vi "SC2 RT.vi"() -> ()   [LabVIEW 2015]
uses:
  SC2 states.ctl
  <vilib>/Platform/TimedLoop/XDataNode/timing_clust.ctl
  <vilib>/Platform/TimedLoop/XDataNode/nitl_modes.ctl
  <vilib>/Platform/TimedLoop/XDataNode/wakeup.ctl
  Encoder bit cluster.ctl
  <vilib>/Platform/TimedLoop/XDataNode/loadnilvce.vi
  <vilib>/Motion/Express/_s/nimc.fb.straightLineMove.startStraightLineMove.axis.modeRelative.0.vi
  <vilib>/Platform/TimedLoop/XDataNode/XDataNode.xnode
  <vilib>/Motion/BlockNode/FB.NIMotion.xnode
  <vilib>/Platform/TimedLoop/XDataNode/XDNodeRunTimeDep.lvlib
  <vilib>/nisyscfg/nisyscfg.lvlib
  <vilib>/nisyscfg/Find Hardware.vi
panel:
  out "Encoder displacement":i32
  in  "Random Sample":bool
  out "Within window?":bool
  in  "Stop":bool
  out "Motor status":bool=TRUE
  in  "Encoder offset":i32=-1277
  in  "Start Sample Change":bool
  out "SC2 State Control":T1=enum."wait"
  out "Encoder readback":errorcluster
  in  "error in (no error)":errorcluster
  out "status":bool
  out "Encoder destination":i32
  in  "New Move (Motor steps)":dbl=10000.0 format="%#_13g"
  in  "New Sample":i16
  in  "Step Window radius":i32=2
  out "Converted Encoder":bool[](array[boolean])
  in  "Motion Resource":refnum<k21>="Axis 1"
  out "Straight Line Move":errorcluster
  out "Raw Encoder":bool[](array[boolean])
  out "Encoder rotation":u16(graph)
  out "Encoder Position":i32
  # "Encoder offset required to \n\"line up\" encoder with wheel.\nSample 64 is -1021 encoder steps\n (or +15362 steps) from the \nencoder's zero point.. Note: Sample \nand encoder numbering run in \nopposite directions"
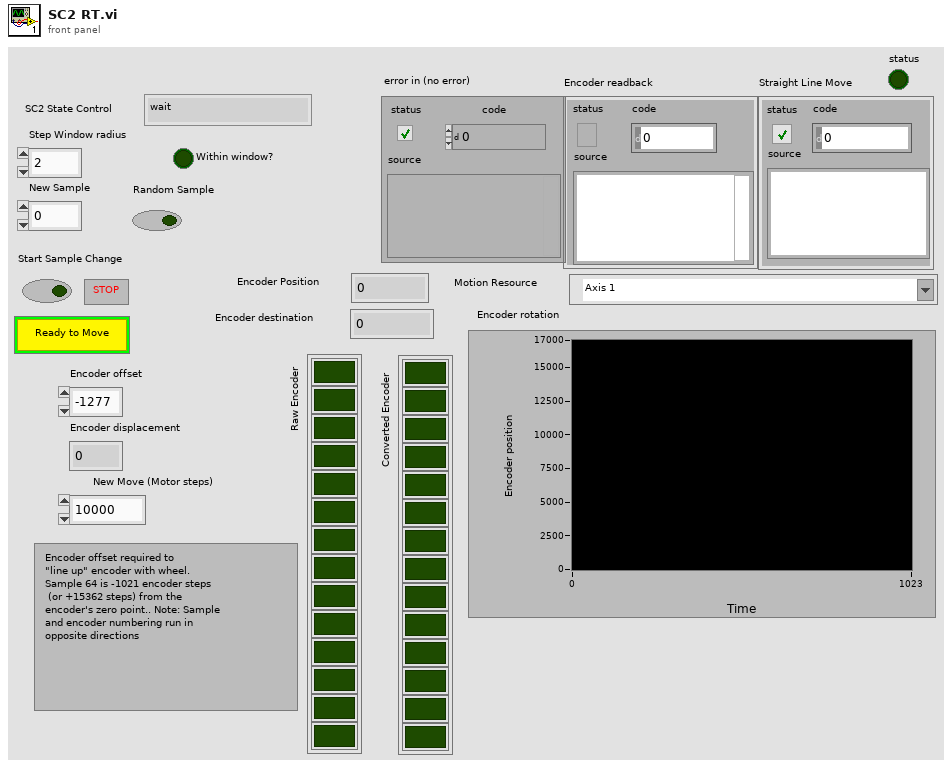
[diagram p1: front panel]
types:
  T1 = typedef "SC2 states.ctl" = enum16{"initialize", "wait", "check position", "rotate wheel", "rotate complete"}
  T2 = typedef "XDNodeRunTimeDep.lvlib/timing_clust.ctl" = cluster{"Expected End [f-1]":u64, "Actual End [f-1]":u64, "Finished Late? [f-1]":bool, "Expected End [i-1]":u64, "Actual End [i-1]":u64, "Finished Late? [i-1]":bool, "Expected Start [i]":u64, "Actual Start [i]":u64, "Expected Start [f]":u64, "Actual Start [f]":u64, "Source Name":string, "Structure Name":string, "Period":i64, "Deadline":i64, "Offset":i64, "Start":i64, "Priority":i32, "Timeout":i32, "Mode":T3, "Wakeup Reason":T4, "Error":errorcluster, "Source Type":string, "Secondary Source Type":string, "Global End Time":u64, "Global Start Time":u64, "Frame Duration":u64, "Iteration Duration":u64, "Assigned CPU":i32, "I/O Scan Engine Mode":u32}
  T3 = typedef "XDNodeRunTimeDep.lvlib/nitl_modes.ctl" = enum32{"No Change", "Process missed periods, maintain original phase", "Discard missed periods, maintain original phase", "Process missed periods, ignore original phase", "Discard missed periods, ignore original phase"}
  T4 = typedef "XDNodeRunTimeDep.lvlib/wakeup.ctl" = enum32{"Normal", "Aborted", "Asynchronous wakeup", "Timing source error", "Timed loop error", "Timeout"}
  T5 = typedef "Encoder bit cluster.ctl" = cluster{"MSB":bool, "13th bit":bool, "12th bit":bool, "11th bit":bool, "10th bit":bool, "9th bit":bool, "8th bit":bool, "7th bit":bool, "6th bit":bool, "5th bit":bool, "4th bit":bool, "3rd bit":bool, "2nd bit":bool, "LSB":bool}
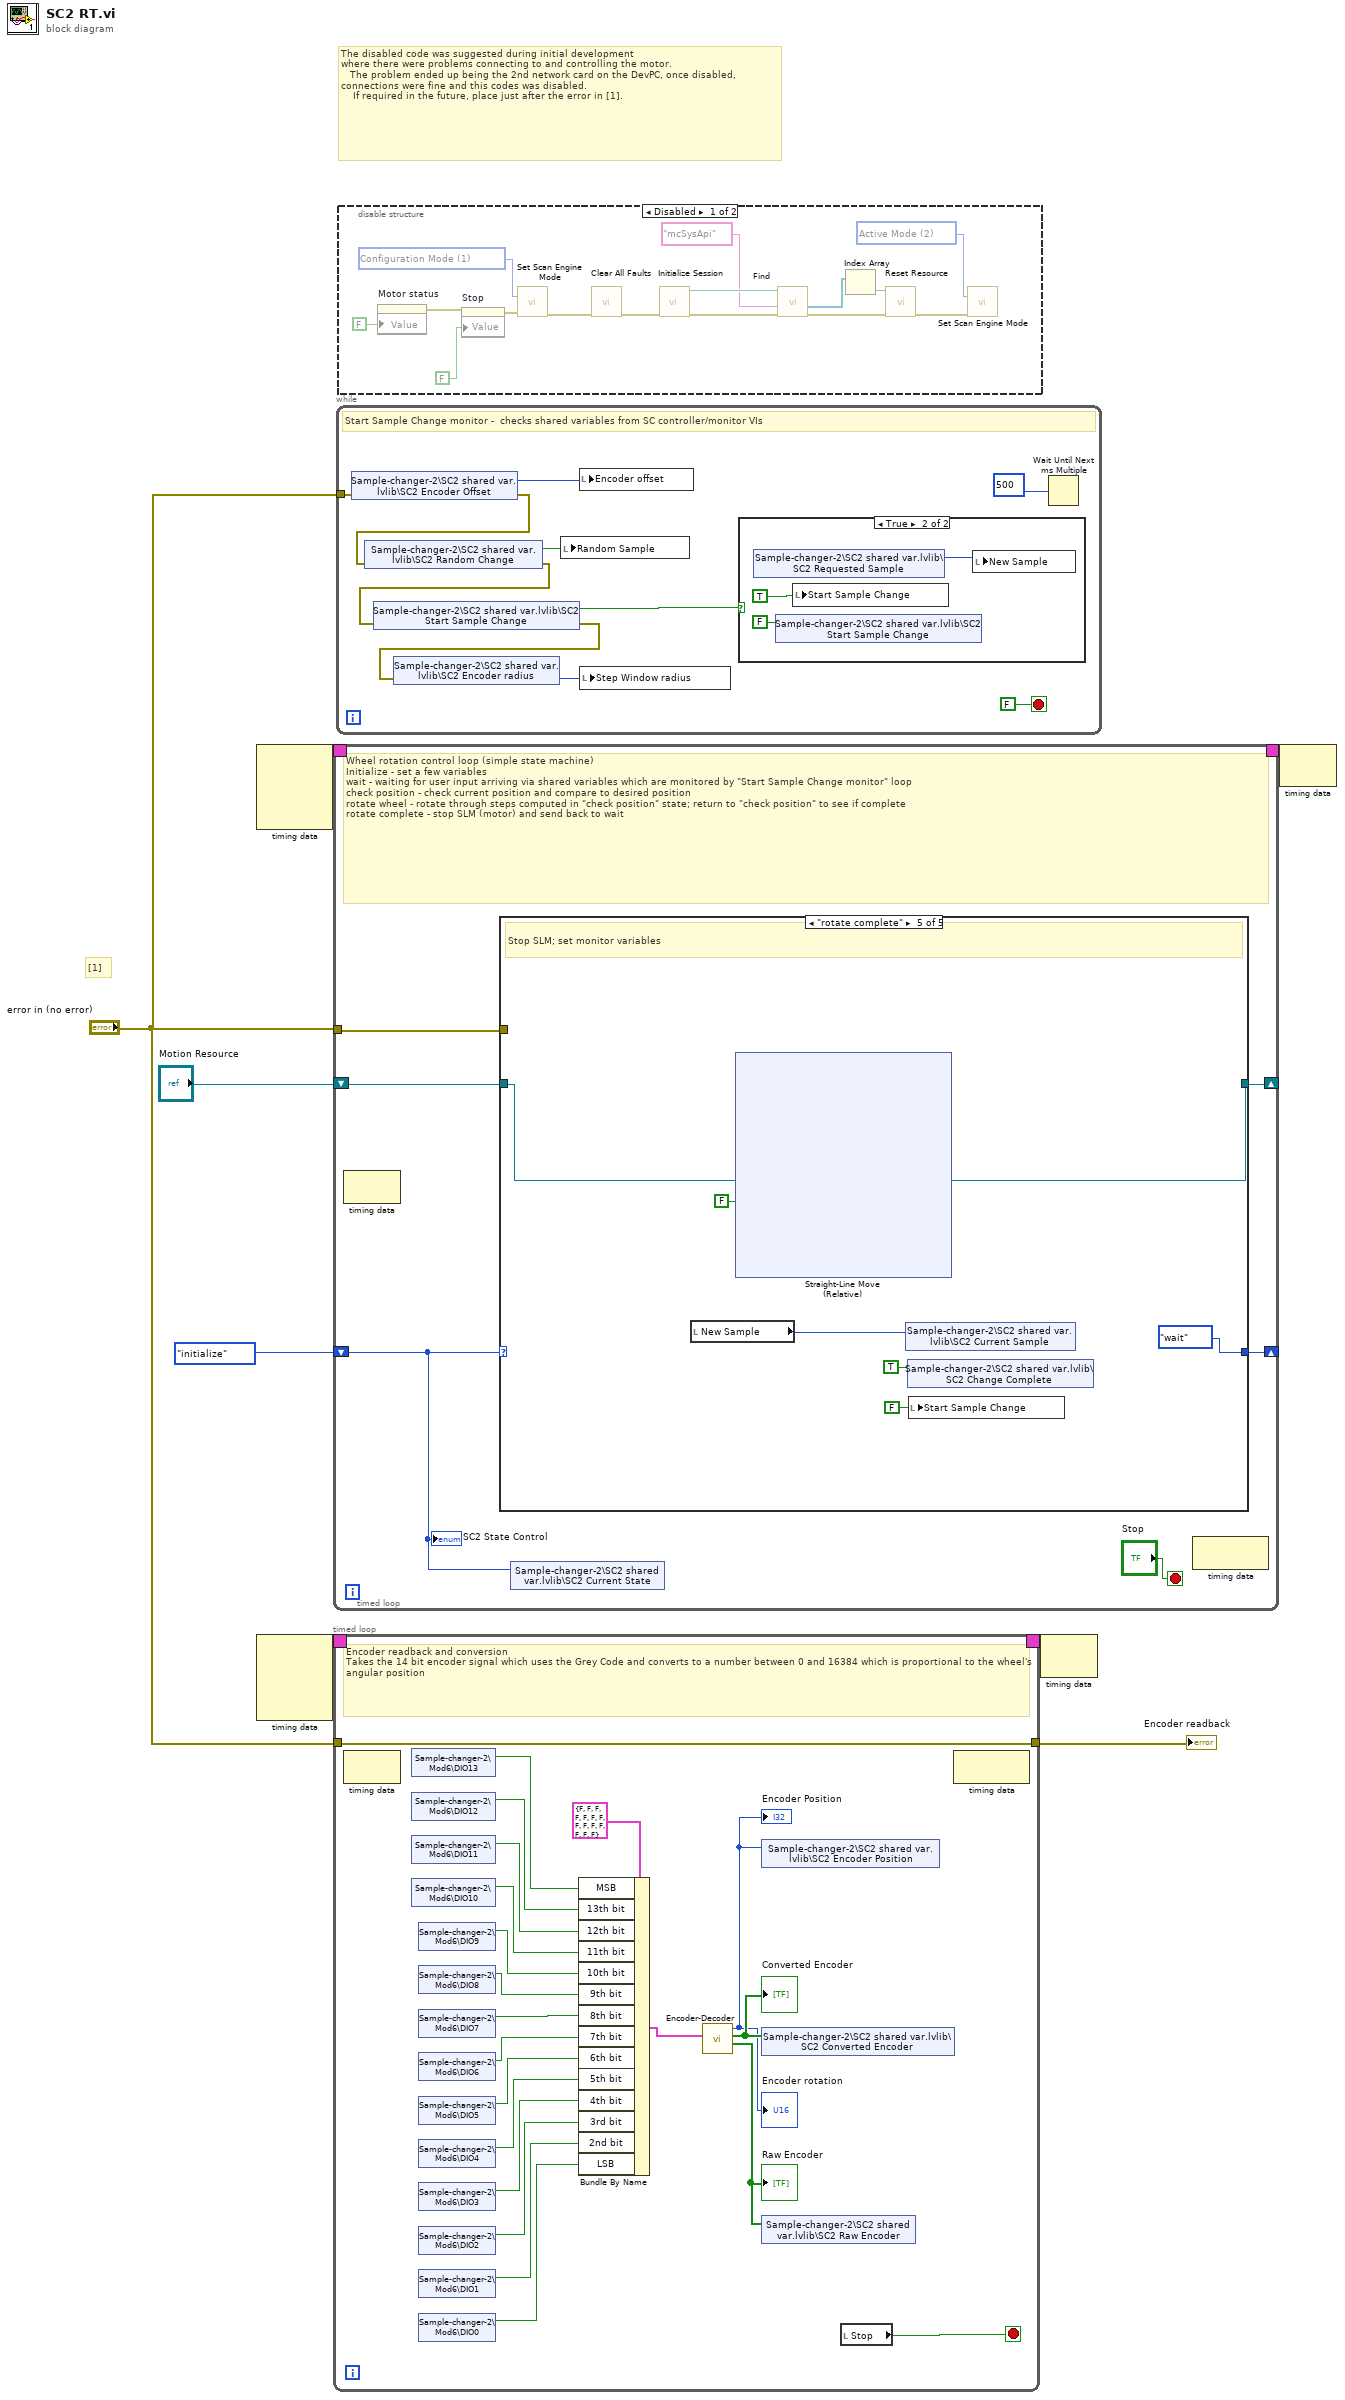
[diagram p0: block diagram]
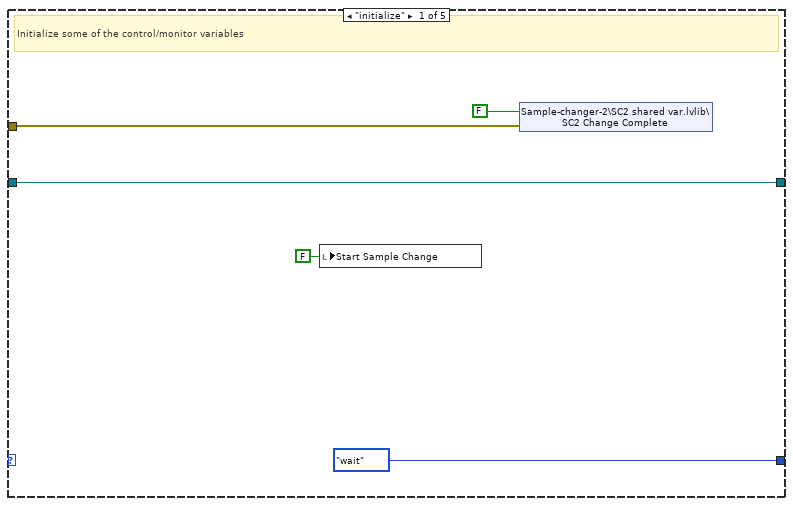
[diagram p4: hidden frame]
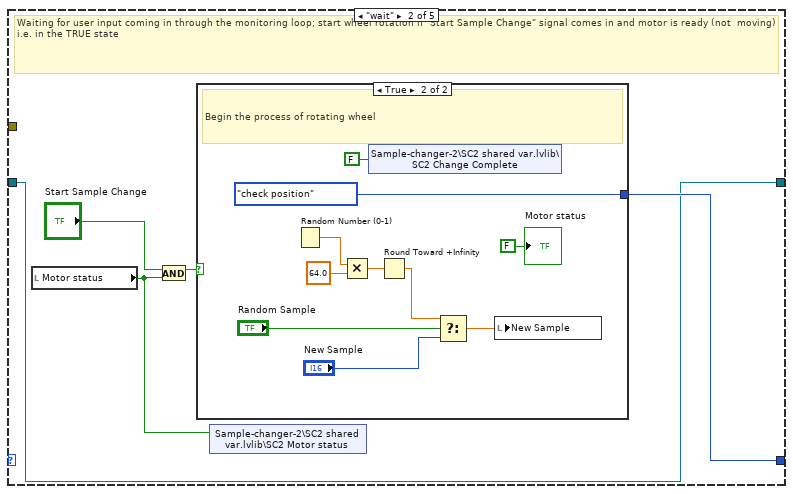
[diagram p5: hidden frame]
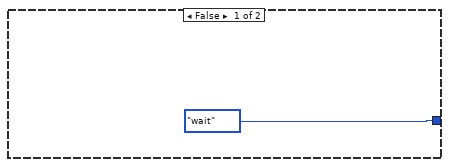
[diagram p6: hidden frame]
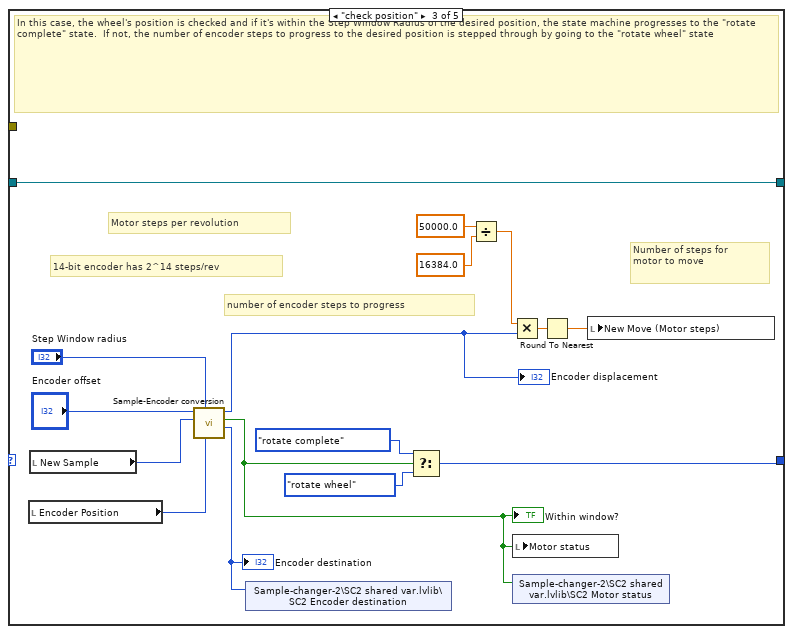
[diagram p7: hidden frame]
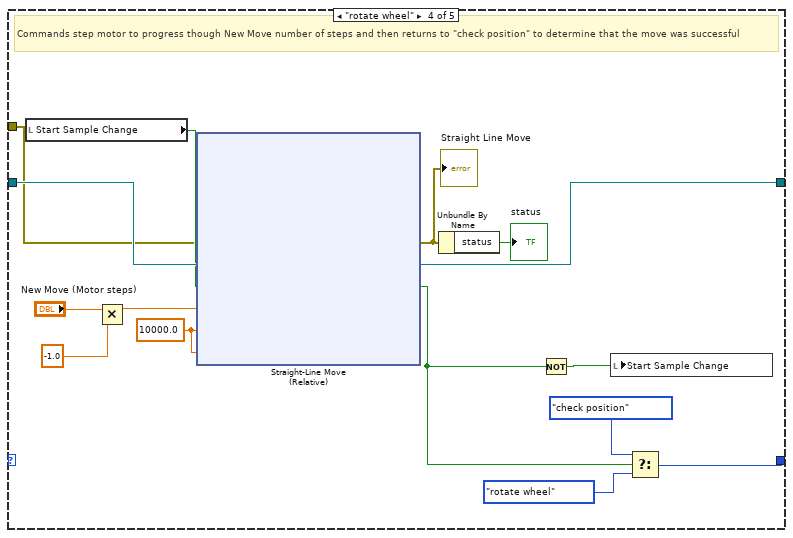
[diagram p8: hidden frame]
diagram:
  # "[1]"
  # "The disabled code was suggested during initial development\nwhere there were problems connecting to and controlling the motor.\n   The problem ended up being the 2nd network card on the DevPC, once disabled, connections were fine and this codes was disabled.  \n    If required in the future, place just after the error in [1]."
  n1 = node-c288() -> (w6:T2)  [unwired: 4 in]
  n2 = node-c288() -> (w8:T2)  [unwired: 4 in]
  n3 = timed-loop {
    timing: w6 -> [_]
    timing-out: [_] -> w5
    shift-right: [w13] -> _
    shift-left: SC2_states."initialize" -> [w9]
    shift-right: [w11] -> _
    shift-left: "Motion Resource" -> [w14]
    tunnel: "error in (no error)" -> [w10]
    stop <- "Stop" stop-if-true
    # "Wheel rotation control loop (simple state machine)\nInitialize - set a few variables \nwait - waiting for user input arriving via shared variables which are monitored by \"Start Sample Change monitor\" loop\ncheck position - check current position and compare to desired position \nrotate wheel - rotate through steps computed in \"check position\" state; return to \"check position\" to see if complete\nrotate complete - stop SLM (motor) and send back to wait"
    n4 = node-c288() -> ()  [unwired: 1 in, 1 out]
    n5 = case shown="\"rotate complete\"" w9 {
      tunnel: w14 -> [w18 w22 w38 w65 w90]
      tunnel: [SC2_states."wait" w23 w51 w60 SC2_states."wait"] -> w13
      tunnel: [w18 w22 w38 w57 w87] -> w11
      tunnel: w10 -> [w15 _ _ w53 _]
      frame "initialize" {
        # "Initialize some of the control/monitor variables"
        n6 = local write "Start Sample Change"(FALSE ("Start Sample Change")) -> ()
        n7 = shared-variable "Sample-changer-2\\SC2 shared var.lvlib\\SC2 Change Complete"(FALSE ("SC2 Change Complete"), error in=w15) -> ()  [unwired: 1 out]
      }
      frame "wait" {
        # "Waiting for user input coming in through the monitoring loop; start wheel rotation if \"Start Sample Change\" signal comes in and motor is ready (not  moving) i.e. in the TRUE state"
        n8 = local read "Motor status"() -> (w20:bool)
        n9 = And(x="Start Sample Change", y=w20) -> (x .and. y?=w21:bool)
        n10 = case shown="True" w21 {
          tunnel: [SC2_states."wait" SC2_states."check position"] -> w23
          frame False {
          }
          frame True {
            # "Begin the process of rotating wheel"
            n11 = Random Number (0-1)() -> (number: 0 to 1=w34:dbl)
            n12 = Multiply(x=w34, y=64.0) -> (x*y=w35:dbl)
            n13 = shared-variable "Sample-changer-2\\SC2 shared var.lvlib\\SC2 Change Complete"(FALSE) -> ()  [unwired: 1 in, 1 out]
            n14 = Round Toward +Infinity(x=w35) -> (ceil(x): smallest int >= x=w29:dbl)
            n15 = Select(t=w29, s="Random Sample", f="New Sample") -> (s? t:f=w28:dbl)
            n16 = local write "New Sample"(w28) -> ()
            "Motor status" <- FALSE ("Motor status")
          }
        }
        n17 = shared-variable "Sample-changer-2\\SC2 shared var.lvlib\\SC2 Motor status"(w20) -> ()  [unwired: 1 in, 1 out]
      }
      frame "check position" {
        # "Number of steps for\nmotor to move"
        # "number of encoder steps to progress"
        # "14-bit encoder has 2^14 steps/rev"
        # "Motor steps per revolution"
        # "In this case, the wheel's position is checked and if it's within the Step WIndow Radius of the desired position, the state machine progresses to the \"rotate complete\" state.  If not, the number of encoder steps to progress to the desired position is stepped through by going to the \"rotate wheel\" state"
        n18 = local read "Encoder Position"() -> (w45:i32)
        n19 = local read "New Sample"() -> (w37:i16)
        n20 = call "Sample-Encoder conversion.vi"("Encoder Position"=w45, "Step Window radius"="Step Window radius", "New Sample Number"=w37, "Encoder offset"="Encoder offset") -> ("Encoder destination"=w43:i32, "Within Range?"=w36:bool, "Encoder displacement"=w46:i32)  [unwired: 5 in]
        "Encoder destination" <- w43
        "Within window?" <- w36
        "Encoder displacement" <- w46
        n21 = shared-variable "Sample-changer-2\\SC2 shared var.lvlib\\SC2 Encoder destination"(w43) -> ()  [unwired: 1 in, 1 out]
        n22 = Select(t=SC2_states."rotate complete", s=w36, f=SC2_states."rotate wheel") -> (s? t:f=w51:T1)
        n23 = Divide(x=50000.0, y=16384.0) -> (x/y=w50:dbl)
        n24 = Multiply(x=w50, y=w46) -> (x*y=w47:dbl)
        n25 = local write "Motor status"(w36) -> ()
        n26 = shared-variable "Sample-changer-2\\SC2 shared var.lvlib\\SC2 Motor status"(w36) -> ()  [unwired: 1 in, 1 out]
        n27 = Round To Nearest(number=w47) -> (nearest integer value=w40:dbl)
        n28 = local write "New Move (Motor steps)"(w40) -> ()
      }
      frame "rotate wheel" {
        w66 = 10000.0
        # "Commands step motor to progress though New Move number of steps and then returns to \"check position\" to determine that the move was successful"
        n29 = local read "Start Sample Change"() -> (w61:bool)
        n30 = Multiply(x="New Move (Motor steps)", y=-1.0) -> (x*y=w56:dbl)
        n31 = xnode "Straight-Line Move\n(Relative)"("error in"=w53, "resource"=w65, "execute"=w61, "position"=w56, "velocity"=w66, "acceleration"=w66) -> ("error out"=w54:errorcluster, "resource out"=w57:refnum<k21>, "done"=w58:bool)
        "Straight Line Move" <- w54
        n32 = Unbundle By Name(w54) -> ("status"=→"status":bool)
        n33 = Not(x=w58) -> (.not. x?=w52:bool)
        n34 = local write "Start Sample Change"(w52) -> ()
        n35 = Select(t=SC2_states."check position", s=w58, f=SC2_states."rotate wheel") -> (s? t:f=w60:T1)
      }
      frame "rotate complete" {
        # "Stop SLM; set monitor variables"
        n36 = local read "New Sample"() -> (w85:i16)
        n37 = xnode "Straight-Line Move\n(Relative)"("resource"=w90, "execute"=FALSE) -> ("resource out"=w87:refnum<k21>)  [unwired: 4 in, 2 out]
        n38 = shared-variable "Sample-changer-2\\SC2 shared var.lvlib\\SC2 Current Sample"(w85) -> ()  [unwired: 1 in, 1 out]
        n39 = shared-variable "Sample-changer-2\\SC2 shared var.lvlib\\SC2 Change Complete"(TRUE ("SC2 Change Complete")) -> ()  [unwired: 1 in, 1 out]
        n40 = local write "Start Sample Change"(FALSE ("Start Sample Change")) -> ()
      }
    }
    n41 = shared-variable "Sample-changer-2\\SC2 shared var.lvlib\\SC2 Current State"(w9) -> ()  [unwired: 1 in, 1 out]
    n42 = node-c288() -> ()  [unwired: 1 in, 1 out]
    "SC2 State Control" <- w9
  }
  n43 = timed-loop {
    timing: w8 -> [_]
    timing-out: [_] -> w7
    tunnel: "error in (no error)" -> [w127]
    tunnel: [w127] -> w2
    stop <- w110 stop-if-true
    # "Encoder readback and conversion\nTakes the 14 bit encoder signal which uses the Grey Code and converts to a number between 0 and 16384 which is proportional to the wheel's angular position"
    n44 = node-c288() -> ()  [unwired: 1 in, 1 out]
    n45 = shared-variable "Sample-changer-2\\Mod6\\DIO13"() -> (w126:bool)  [unwired: 1 in, 1 out]
    n46 = shared-variable "Sample-changer-2\\Mod6\\DIO12"() -> (w125:bool)  [unwired: 1 in, 1 out]
    n47 = shared-variable "Sample-changer-2\\Mod6\\DIO11"() -> (w124:bool)  [unwired: 1 in, 1 out]
    n48 = shared-variable "Sample-changer-2\\Mod6\\DIO10"() -> (w123:bool)  [unwired: 1 in, 1 out]
    n49 = shared-variable "Sample-changer-2\\Mod6\\DIO9"() -> (w122:bool)  [unwired: 1 in, 1 out]
    n50 = shared-variable "Sample-changer-2\\Mod6\\DIO8"() -> (w121:bool)  [unwired: 1 in, 1 out]
    n51 = shared-variable "Sample-changer-2\\Mod6\\DIO7"() -> (w120:bool)  [unwired: 1 in, 1 out]
    n52 = shared-variable "Sample-changer-2\\Mod6\\DIO6"() -> (w119:bool)  [unwired: 1 in, 1 out]
    n53 = shared-variable "Sample-changer-2\\Mod6\\DIO5"() -> (w118:bool)  [unwired: 1 in, 1 out]
    n54 = shared-variable "Sample-changer-2\\Mod6\\DIO4"() -> (w117:bool)  [unwired: 1 in, 1 out]
    n55 = shared-variable "Sample-changer-2\\Mod6\\DIO3"() -> (w116:bool)  [unwired: 1 in, 1 out]
    n56 = shared-variable "Sample-changer-2\\Mod6\\DIO2"() -> (w115:bool)  [unwired: 1 in, 1 out]
    n57 = shared-variable "Sample-changer-2\\Mod6\\DIO1"() -> (w114:bool)  [unwired: 1 in, 1 out]
    n58 = shared-variable "Sample-changer-2\\Mod6\\DIO0"() -> (w113:bool)  [unwired: 1 in, 1 out]
    n59 = Bundle By Name(cluster=T5 {"MSB"=FALSE, "13th bit"=FALSE, "12th bit"=FALSE, "11th bit"=FALSE, "10th bit"=FALSE, "9th bit"=FALSE, "8th bit"=FALSE, "7th bit"=FALSE, "6th bit"=FALSE, "5th bit"=FALSE, "4th bit"=FALSE, "3rd bit"=FALSE, "2nd bit"=FALSE, "LSB"=FALSE} ("Cluster"), "MSB"=w126, "13th bit"=w125, "12th bit"=w124, "11th bit"=w123, "10th bit"=w122, "9th bit"=w121, "8th bit"=w120, "7th bit"=w119, "6th bit"=w118, "5th bit"=w117, "4th bit"=w116, "3rd bit"=w115, "2nd bit"=w114, "LSB"=w113) -> (w111:T5)
    n60 = call "Encoder-Decoder.vi"("Encoder data"=w111) -> ("Raw bits"=w128:bool[], "Converted bits"=w130:bool[], "Encoder position"=w129:u16)  [unwired: 8 in]
    "Encoder Position" <- w129
    "Encoder rotation" <- w129
    "Raw Encoder" <- w128
    "Converted Encoder" <- w130
    n61 = shared-variable "Sample-changer-2\\SC2 shared var.lvlib\\SC2 Encoder Position"(w129) -> ()  [unwired: 1 in, 1 out]
    n62 = shared-variable "Sample-changer-2\\SC2 shared var.lvlib\\SC2 Converted Encoder"(w130) -> ()  [unwired: 1 in, 1 out]
    n63 = shared-variable "Sample-changer-2\\SC2 shared var.lvlib\\SC2 Raw Encoder"(w128) -> ()  [unwired: 1 in, 1 out]
    n64 = local read "Stop"() -> (w110:bool)
    n65 = node-c288() -> ()  [unwired: 1 in, 1 out]
  }
  "Encoder readback" <- w2
  n66 = while {
    tunnel: "error in (no error)" -> [w133]
    stop <- FALSE stop-if-true
    # "Start Sample Change monitor -  checks shared variables from SC controller/monitor VIs"
    n67 = shared-variable "Sample-changer-2\\SC2 shared var.lvlib\\SC2 Encoder Offset"(error in=w133) -> (w139:i16, error out=w138:errorcluster)
    n68 = shared-variable "Sample-changer-2\\SC2 shared var.lvlib\\SC2 Random Change"(error in=w138) -> (w136:bool, error out=w137:errorcluster)
    n69 = shared-variable "Sample-changer-2\\SC2 shared var.lvlib\\SC2 Start Sample Change"(error in=w137) -> (w142:bool, error out=w134:errorcluster)
    n70 = shared-variable "Sample-changer-2\\SC2 shared var.lvlib\\SC2 Encoder radius"(error in=w134) -> (w135:i32)  [unwired: 1 out]
    n71 = local write "Random Sample"(w136) -> ()
    n72 = local write "Encoder offset"(w139) -> ()
    n73 = local write "Step Window radius"(w135) -> ()
    n74 = case shown="True" w142 {
      frame False {
      }
      frame True {
        n75 = shared-variable "Sample-changer-2\\SC2 shared var.lvlib\\SC2 Requested Sample"() -> (w144:u8)  [unwired: 1 in, 1 out]
        n76 = shared-variable "Sample-changer-2\\SC2 shared var.lvlib\\SC2 Start Sample Change"(FALSE ("Start Sample Change")) -> ()  [unwired: 1 in, 1 out]
        n77 = local write "Start Sample Change"(TRUE ("Start Sample Change")) -> ()
        n78 = local write "New Sample"(w144) -> ()
      }
    }
    n79 = Wait Until Next ms Multiple(millisecond multiple=500) -> ()  [unwired: 1 out]
  }
  n80 = disable-structure shown="Disabled" {
    frame Disabled {
      w152 = 2 items=["Configuration Mode"=1, "Active Mode"=2] ("mode (Active Mode)")
      w154 = 1 items=["Configuration Mode"=1, "Active Mode"=2] ("mode (Active Mode)")
      n81 = property on="Motor status" class="Bool (strict)"("Value"=FALSE ("Motor status")) -> (error out=w146:errorcluster)  [unwired: 2 in, 1 out]
      n82 = property on="Stop" class="Bool (strict)"(error in=w146, "Value"=FALSE ("Stop")) -> (error out=w148:errorcluster)  [unwired: 1 in, 1 out]
      n83 = call <vilib>:"Set Scan Engine Mode.vi"("mode (Active Mode)"=w154, "error in (no error)"=w148) -> ("error out"=w151:errorcluster)  [unwired: 13 in]
      n84 = call <vilib>:"Clear All Faults.vi"("error in (no error)"=w151) -> ("error out"=w158:errorcluster)  [unwired: 10 in]
      n85 = call <vilib>:"Initialize Session.vi"("error in (no error)"=w158) -> ("error out"=w159:errorcluster, "Session out"=w160:refnum<k21>)  [unwired: 9 in]
      n86 = call-poly <vilib>:"Find.vi"("error in (no error)"=w159, "Experts"="mcSysApi" ("experts"), "Session in"=w160) -> ("error out"=w150:errorcluster, "Resources out"=w156:refnum<k20>[])  [unwired: 5 in, 2 out]
      n87 = Index Array(array=w156) -> (element=w157:refnum<k20>)  [unwired: 1 in]
      n88 = call <vilib>:"Reset Resource.vi"("error in (no error)"=w150, "Resource in"=w157) -> ("error out"=w153:errorcluster)  [unwired: 6 in, 3 out]
      n89 = call <vilib>:"Set Scan Engine Mode.vi"("mode (Active Mode)"=w152, "error in (no error)"=w153) -> ()  [unwired: 13 in, 1 out]
    }
    frame Enabled {
    }
  }
  n90 = node-c288(w7) -> ()  [unwired: 1 out]
  n91 = node-c288(w5) -> ()  [unwired: 1 out]
